vi "CLD 16 Add process.vi"(8 "Fehler (Eingang, kein Fehler)":errorcluster, 11 "Cluster (Eingang)":T1 {"Statusanzeige"."Prozesswert" format="%#.3g"}) -> (0 "Fehler (Ausgang)":errorcluster, 3 "Cluster (Ausgang)":T1 {"Statusanzeige"."Prozesswert" format="%#.3g"})   [LabVIEW 2009]
doc: "CLD-Übung 16\n\nDieses SubVI simuliert die Verarbeitungsanforderungen und wird aufgerufen, wenn die Schaltfläche \"Verwenden\" gedrückt wird. Das SubVI enthält eine kurze Verzögerung. Während dieser Zeit wird die Verwenden-Schaltfläche deaktiviert wird."
uses:
  CLD 16 Control Panel.ctl
  CLD 16 Status Panel.ctl
  CLD 16 Data Cluster.ctl
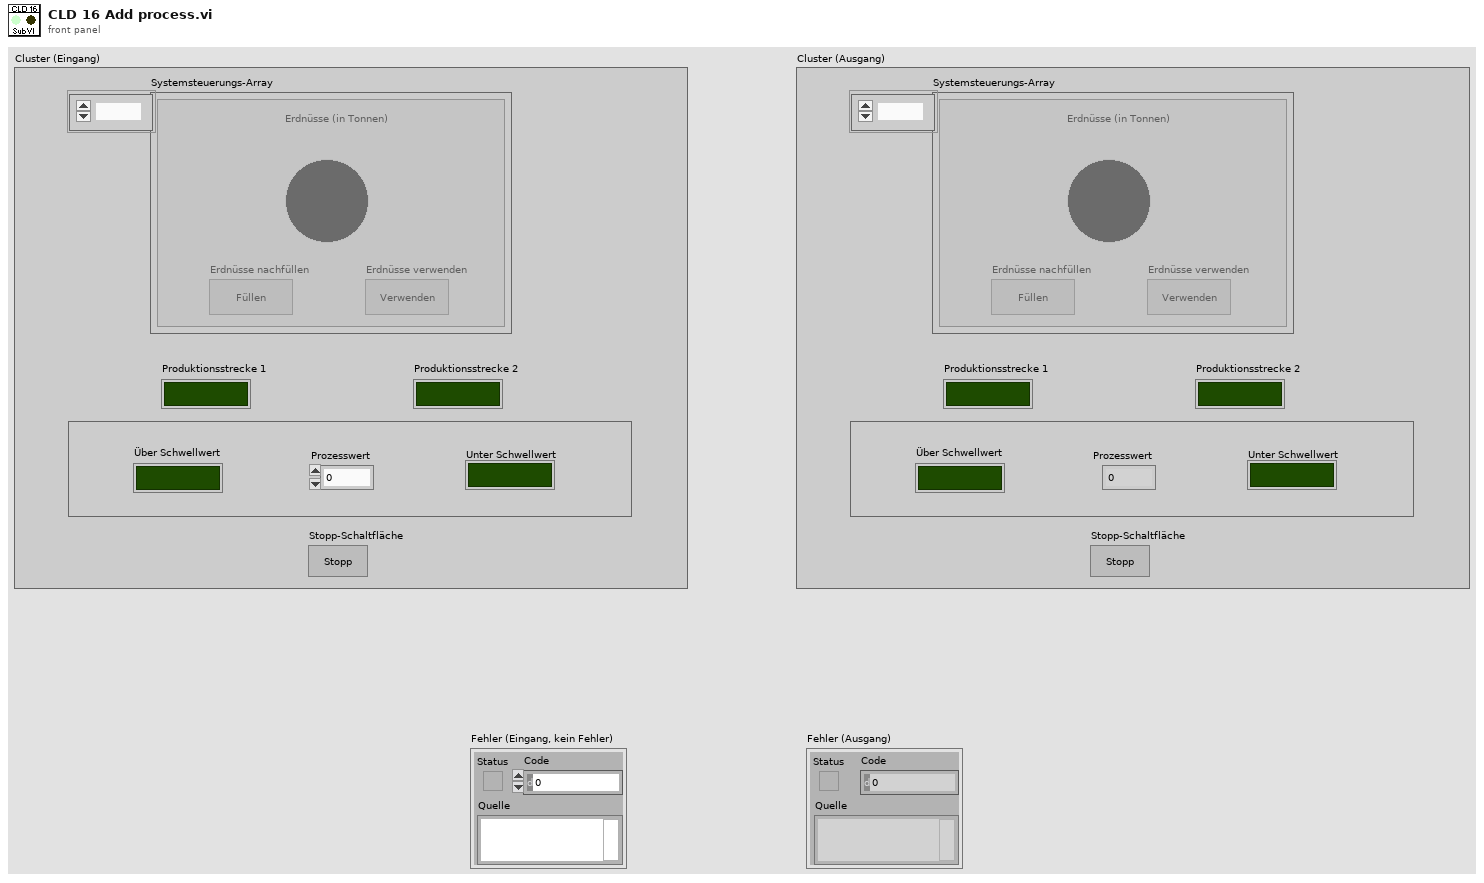
[diagram p1: front panel]
types:
  T1 = typedef "CLD 16 Data Cluster.ctl" = cluster{"Systemsteuerungs-Array":T2[], "Statusanzeige":T3, "Produktionsstrecke 1":bool, "Produktionsstrecke 2":bool, "Stopp-Schaltfläche":bool}
  T2 = typedef "CLD 16 Control Panel.ctl" = cluster{"Erdnüsse (in Tonnen)":i8, "Erdnüsse nachfüllen":bool, "Erdnüsse verwenden":bool}
  T3 = typedef "CLD 16 Status Panel.ctl" = cluster{"Über Schwellwert":bool, "Unter Schwellwert":bool, "Prozesswert":dbl}
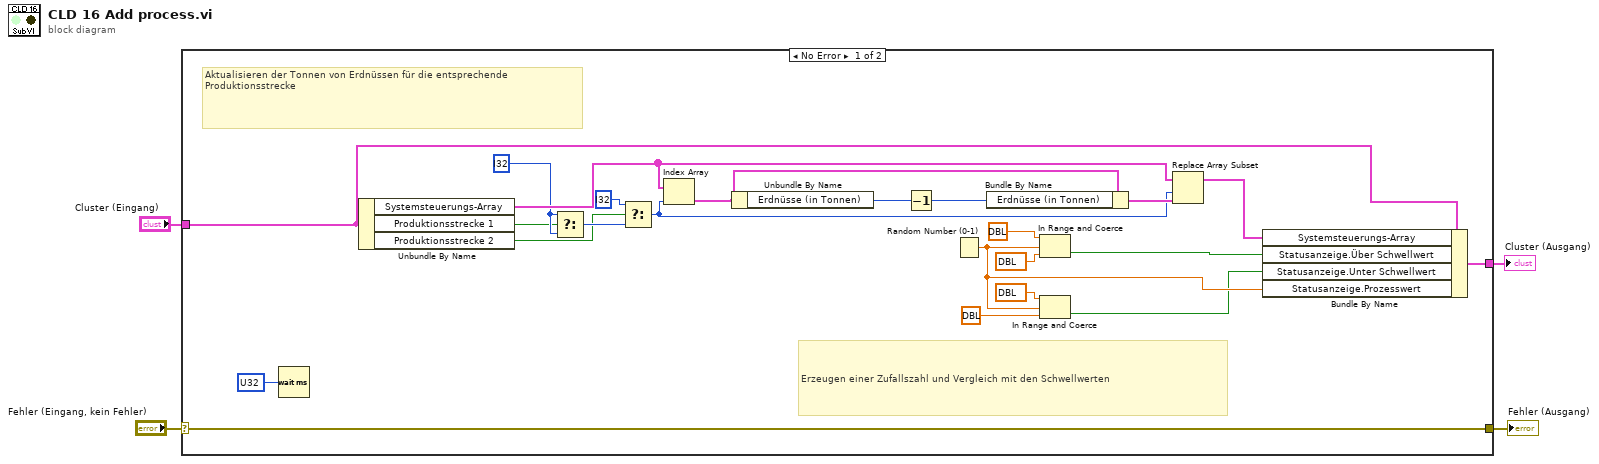
[diagram p0: block diagram]
diagram:
  n1 = case shown="No Error" "Fehler (Eingang, kein Fehler)" {
    selector: "Fehler (Eingang, kein Fehler)" -> [w6 w28]
    tunnel: [w27 w29] -> w4
    tunnel: "Cluster (Eingang)" -> [w25 w29]
    tunnel: [w6 w28] -> w1
    frame #0 {
      w18 = i32 ?
      # "Aktualisieren der Tonnen von Erdnüssen für die entsprechende Produktionsstrecke"
      # "Erzeugen einer Zufallszahl und Vergleich mit den Schwellwerten"
      n2 = Wait (ms)(milliseconds to wait=u32 ? ("Zu wartende ms")) -> ()  [unwired: 1 out]
      n3 = Unbundle By Name(w25) -> ("Systemsteuerungs-Array"=w22:T2[], "Produktionsstrecke 1"=w14:bool, "Produktionsstrecke 2"=w15:bool)
      n4 = Select(t=w18, s=w14, f=w18) -> (s? t:f=w16:i32)
      n5 = Select(t=i32 ?, s=w15, f=w16) -> (s? t:f=w23:i32)
      n6 = Index Array(array=w22, index=w23) -> (element=w19:T2)
      n7 = Unbundle By Name(w19) -> ("Erdnüsse (in Tonnen)"=w20:i8)
      n8 = Decrement(x=w20) -> (x-1=w21:i8)
      n9 = Random Number (0-1)() -> (number: 0 to 1=w9:dbl)
      n10 = Bundle By Name(cluster=w19, "Erdnüsse (in Tonnen)"=w21) -> (w24:T2)
      n11 = In Range and Coerce(upper limit=dbl ? ("Obergrenze"), x=w9, lower limit=dbl ? ("Untergrenze")) -> (In Range?=w8:bool)  [unwired: 1 out]
      n12 = In Range and Coerce(upper limit=dbl ? ("Obergrenze"), x=w9, lower limit=dbl ? ("Untergrenze")) -> (In Range?=w7:bool)  [unwired: 1 out]
      n13 = Replace Array Subset(array=w22, new element=w24, index=w23) -> (w26:T2[])
      n14 = Bundle By Name(cluster=w25, "Systemsteuerungs-Array"=w26, "Statusanzeige.Über Schwellwert"=w8, "Statusanzeige.Unter Schwellwert"=w7, "Statusanzeige.Prozesswert"=w9) -> (w27:T1)
    }
    frame #1 {
    }
  }
  "Cluster (Ausgang)" <- w4
  "Fehler (Ausgang)" <- w1
